vi "Sensor.vi"(8 "error in (no error)":errorcluster) -> (0 "error out":errorcluster)   [LabVIEW 2010]
doc: "This VI is an abstraction between the hardware and the simulation"
uses:
  Database/DB_control.ctl
  Controller/Hardware_Enum.ctl
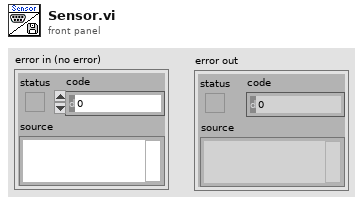
[diagram p1: front panel]
types:
  T1 = typedef "Hardware_Enum.ctl" = enum16{"Simulation", "Hardware"}
  T2 = typedef "DB_control.ctl" = enum16{"Initi_FGV", "Open", "Get_Data", "Write_Data", "Write_File", "Close_File"}
  T3 = typedef "DB_Data.ctl" = cluster{"Door Open Time":dbl, "Travel Time":dbl, "Inactivity Time":dbl, "Door Close Time ":dbl, "Hardware Bit Sensor":T1, "Hardware Bit User console":T1, "Hardware Bit Display":T1, "Controller Bit Display":T1}
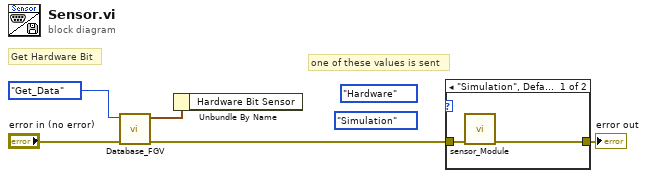
[diagram p0: block diagram]
diagram:
  (unwired) Hardware_Enum."Hardware" ("Hardware Bit")
  (unwired) Hardware_Enum."Simulation" ("Hardware Bit")
  # "one of these values is sent"
  # "Get Hardware Bit"
  n1 = call "Database_FGV.vi"("error in (no error)"="error in (no error)", "DB Control"=DB_control."Get_Data") -> ("error out"=w2:errorcluster, "DB Data Out"=w1:T3)  [unwired: 8 in]
  n2 = Unbundle By Name(w1) -> ()  [unwired: 1 out]
  n3 = case shown="\"Simulation\", Default" {
    selector: _ -> [_ _]
    tunnel: [w6 w8] -> w3
    tunnel: w2 -> [w7 w8]
    frame "Simulation", Default {
      n4 = call "sensor_Module.vi"("error in (no error)"=w7) -> ("error out"=w6:errorcluster)  [unwired: 10 in]
    }
    frame "Hardware" {
      # "Hardware VI TBD"
    }
  }
  "error out" <- w3
